vi "Omron TCP FINS-Write Data(I16 Array).vi"(8 "error in":errorcluster, 9 "Data":i16[](array[numeric]), 10 "Write Setting(I16 Array)":T1={"I/O Memory Address"=130, "Beginning Address"=0} {"I/O Memory Address" items=["DM"=130, "CIO"=176, "WR"=177, "HR"=178, "AR"=179, "TIM"=137, "EM"=152]}, 11 "Buffer Data In":T2) -> (0 "error out":errorcluster, 3 "Buffer Data Out":T2)   [LabVIEW 2016]
uses:
  Data Def/Omron TCP FINS-Buffer Data.ctl
  Data Def/Omron TCP FINS-Command Code.ctl
  Data Def/Omron TCP FINS-FINS Command Frame.ctl
  Data Def/Omron TCP FINS-Memory Area Write Data.ctl
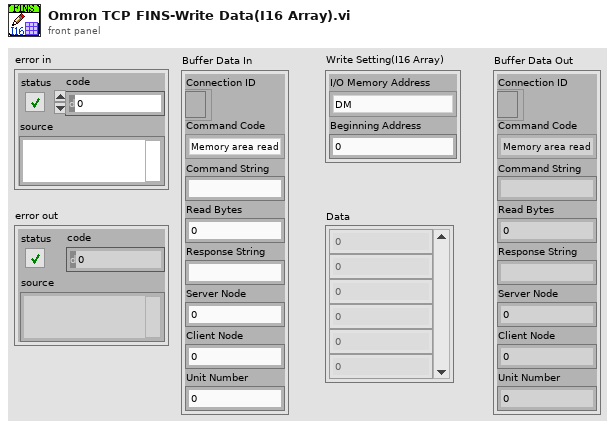
[diagram p1: front panel]
types:
  T1 = cluster{"I/O Memory Address":u8, "Beginning Address":u16}
  T2 = typedef "Omron TCP FINS-Buffer Data.ctl" = cluster{"Connection ID":refnum<k5>, "Command Code":T3, "Command String":string, "Read Bytes":i32, "Response String":string, "Server Node":u8, "Client Node":u8, "Unit Number":u8}
  T3 = typedef "Omron TCP FINS-Command Code.ctl" = enum16{"Memory area read", "Memory area write"}
  T4 = typedef "Omron TCP FINS-Memory Area Write Data.ctl" = cluster{"I/O Memory Address":u8, "Beginning Address":u16, "Data":i16[]}
  T5 = typedef "Omron TCP FINS-FINS Command Frame.ctl" = cluster{"Command Code":T3, "Command Data":variant}
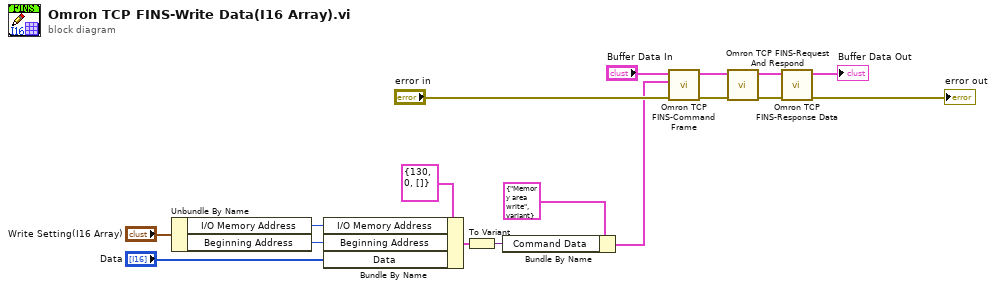
[diagram p0: block diagram]
diagram:
  n1 = Unbundle By Name("Write Setting(I16 Array)") -> ("I/O Memory Address"=w4:u8, "Beginning Address"=w3:u16)
  n2 = Bundle By Name(cluster=T4 {"I/O Memory Address"=130, "Beginning Address"=0, "Data"=[]} ("Memory Area Write Data"), "I/O Memory Address"=w4, "Beginning Address"=w3, "Data"="Data") -> (w6:T4)
  n3 = To Variant(anything=w6) -> (Variant=w15:variant)
  n4 = Bundle By Name(cluster=T5 {"Command Code"=enum."Memory area write", "Command Data"=variant} ("FINS Command Frame"), "Command Data"=w15) -> (w13:T5)
  n5 = call "Omron TCP FINS-Command Frame.vi"("error in"="error in", "FINS Command Frame"=w13, "Buffer Data In"="Buffer Data In") -> ("error out"=w11:errorcluster, "Buffer Data Out"=w12:T2)  [unwired: 7 in]
  n6 = call "Omron TCP FINS-Request And Respond.vi"("error in"=w11, "Buffer Data In"=w12) -> ("error out"=w9:errorcluster, "Buffer Data Out"=w10:T2)  [unwired: 8 in]
  n7 = call "Omron TCP FINS-Response Data.vi"("error in"=w9, "Buffer Data In"=w10) -> ("error out"=→"error out":errorcluster, "Buffer Data Out"=→"Buffer Data Out":T2)  [unwired: 7 in, 1 out]
